vi "max.vi"(10 "Numeric 3":dbl, 11 "Numeric in":sgl) -> (2 "max":sgl)   [LabVIEW 2022 SP3]
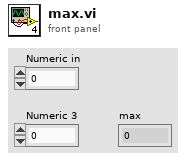
[diagram p1: front panel]
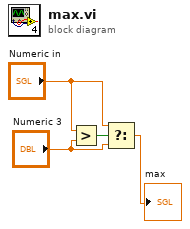
[diagram p0: block diagram]
diagram:
  n1 = Greater?(x="Numeric in", y="Numeric 3") -> (0:w1:bool)
  n2 = Select(t="Numeric in", s=w1, f="Numeric 3") -> (s? t:f=→"max":dbl)
